vi "Autoscroll.vi"(11 "ConsoleView Sink in":refnum<class "ConsoleView.lvclass">) -> (0 "error out":errorcluster, 3 "ConsoleView Sink out":refnum<class "ConsoleView.lvclass">)   [LabVIEW 2017, in "ConsoleView.lvlib" / "ConsoleView.lvclass"]
uses:
  ConsoleView.lvclass
  ConsoleView.lvclass/ConsoleView.ctl
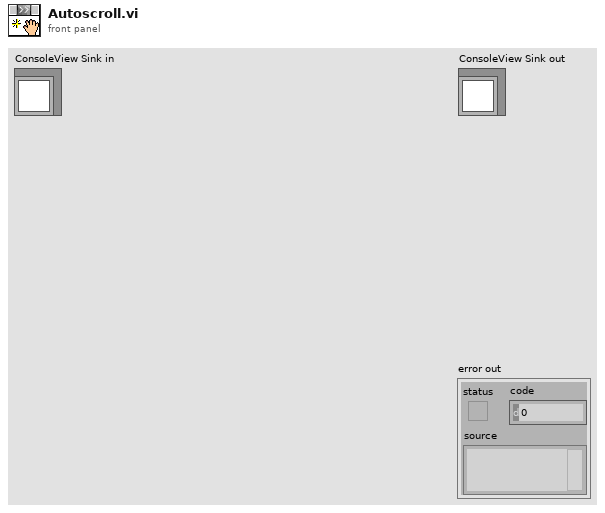
[diagram p1: front panel]
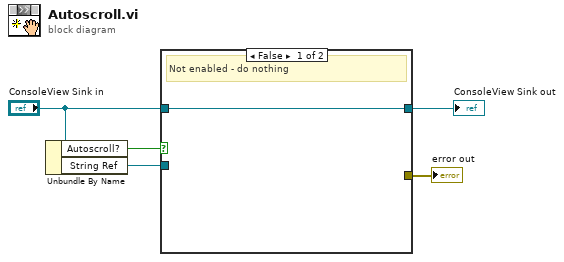
[diagram p0: block diagram]
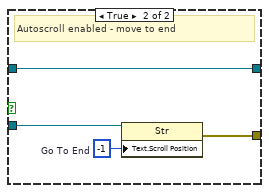
[diagram p2: hidden frame]
diagram:
  n1 = Unbundle By Name("ConsoleView Sink in") -> ("Autoscroll?"=w3:bool, "String Ref"=w2:refnum<vi>)
  n2 = case shown="False" w3 {
    tunnel: [w6 w10] -> w5
    tunnel: "ConsoleView Sink in" -> [w6 w10]
    tunnel: w2 -> [_ w9]
    tunnel: [_ w7] -> w1
    frame False {
      # "Not enabled - do nothing"
    }
    frame True {
      w8 = -1  # Go To End
      # "Autoscroll enabled - move to end"
      n3 = property class="Str"(reference=w9, "Text.Scroll Position"=w8) -> (error out=w7:errorcluster)  [unwired: 1 in, 1 out]
    }
  }
  "error out" <- w1
  "ConsoleView Sink out" <- w5
